vi "ThetaConvertor.vi"(8 "Theta2IN":dbl, 11 "Theta1IN":dbl) -> (0 "Theta1OUT":dbl, 3 "Theta2OUT":dbl)   [LabVIEW 2019]
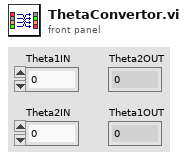
[diagram p1: front panel]
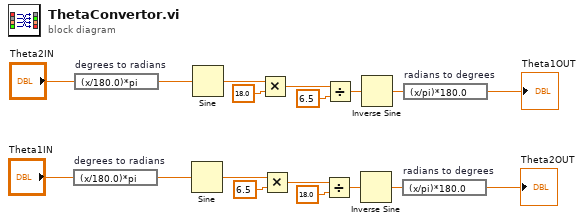
[diagram p0: block diagram]
diagram:
  n1 = expression code="(x/180.0)*pi" "degrees to radians"("Theta1IN") -> (w3:dbl)
  n2 = expression code="(x/180.0)*pi" "degrees to radians"("Theta2IN") -> (w10:dbl)
  n3 = Sine(x=w3) -> (sin(x)=w4:dbl)
  n4 = Sine(x=w10) -> (sin(x)=w11:dbl)
  n5 = Multiply(x=w11, y=18.0) -> (x*y=w13:dbl)
  n6 = Multiply(x=w4, y=6.5) -> (x*y=w6:dbl)
  n7 = Divide(x=w6, y=18.0) -> (x/y=w8:dbl)
  n8 = Divide(x=w13, y=6.5) -> (x/y=w15:dbl)
  n9 = Inverse Sine(1:w8) -> (0:w9:dbl)
  n10 = Inverse Sine(1:w15) -> (0:w16:dbl)
  n11 = expression code="(x/pi)*180.0" "radians to degrees"(w9) -> (→"Theta2OUT":dbl)
  n12 = expression code="(x/pi)*180.0" "radians to degrees"(w16) -> (→"Theta1OUT":dbl)
